vi "Kwang Min IHC images.vi"() -> ()   [LabVIEW 2020]
uses:
  <vilib>/picture/picture.llb/Draw True-Color Pixmap.vi
panel:
  out "SUM":u32
  in  "Find blue\nobjects?":bool
  in  "Count cells?":bool
  out "#cells":u8
  in  "Min cell size":i16=5
  in  "BLUE treshold":u8=175
  in  "GREEN treshold":u8=173
  in  "RED treshold":u8=180
  out "residue":i32
  in  "Binning points":u16=1
  out "BLUE":u8[](array[numeric])
  out "GREEN":u8[](array[numeric])
  out "RED":u8[](array[numeric])
  out "min BLUE":u8
  out "max BLUE":u8
  out "min GREEN":u8
  out "max GREEN":u8
  out "min RED":u8
  out "max RED":u8
  in  "stop":bool
  in  "rect":T1={"left"=38, "top"=68, "right"=53, "bottom"=89}
  in  "subset rect":T1={"left"=0, "top"=0, "right"=100, "bottom"=100}
  out "size(s)":i32[](array[numeric])
  out "new picture":picture
  out "Mask":u8[][](graph)
  in  "path to JPEG file":path
  # "cyan\nparticles"
  # "red\nparticles"
  # "All"
  # "210\n240\n165"
  # "240\n245\n250"
  # "0\n255\n255"
  # "170\n163\n183"
  # "159-255\n153-236\n175-242"
  # "926x1716"
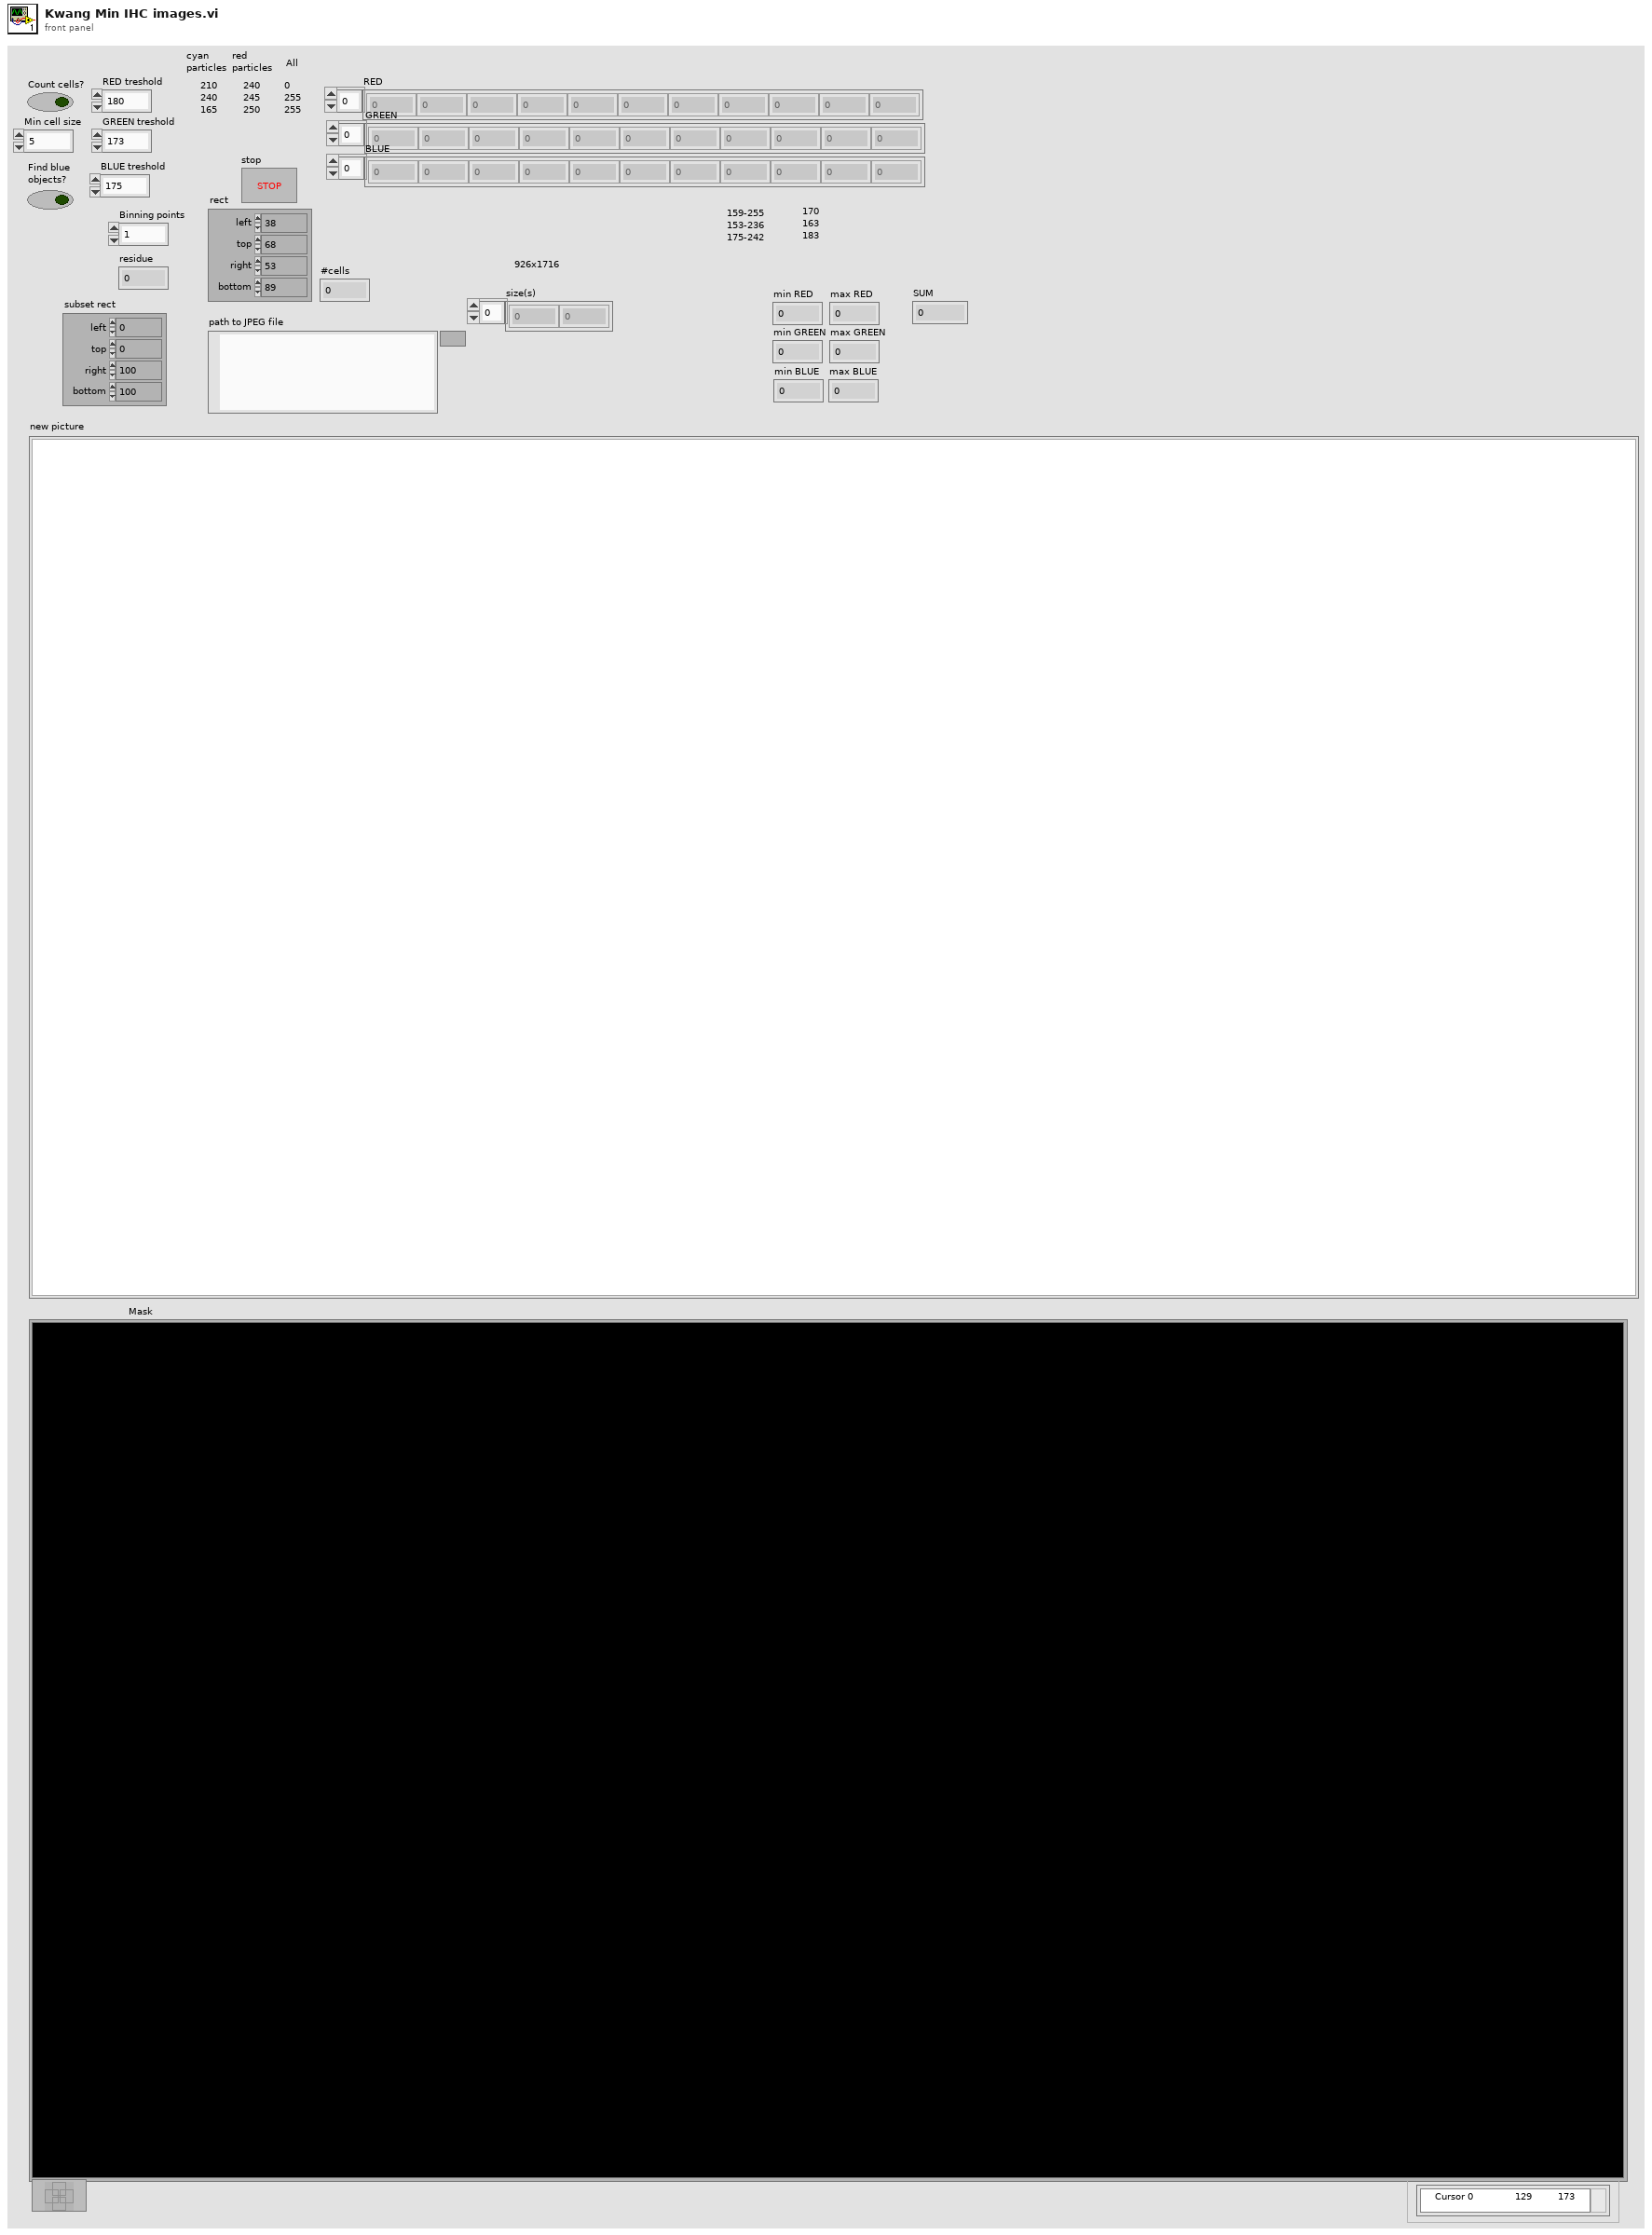
[diagram p1: front panel]
types:
  T1 = cluster{"left":i16, "top":i16, "right":i16, "bottom":i16}
  T2 = typedef "imagedata.ctl" = cluster{"image type":i32, "image depth":i32, "image":u8[], "mask":u8[], "colors":u32[], "Rectangle":cluster{"left":i16, "top":i16, "right":i16, "bottom":i16}}
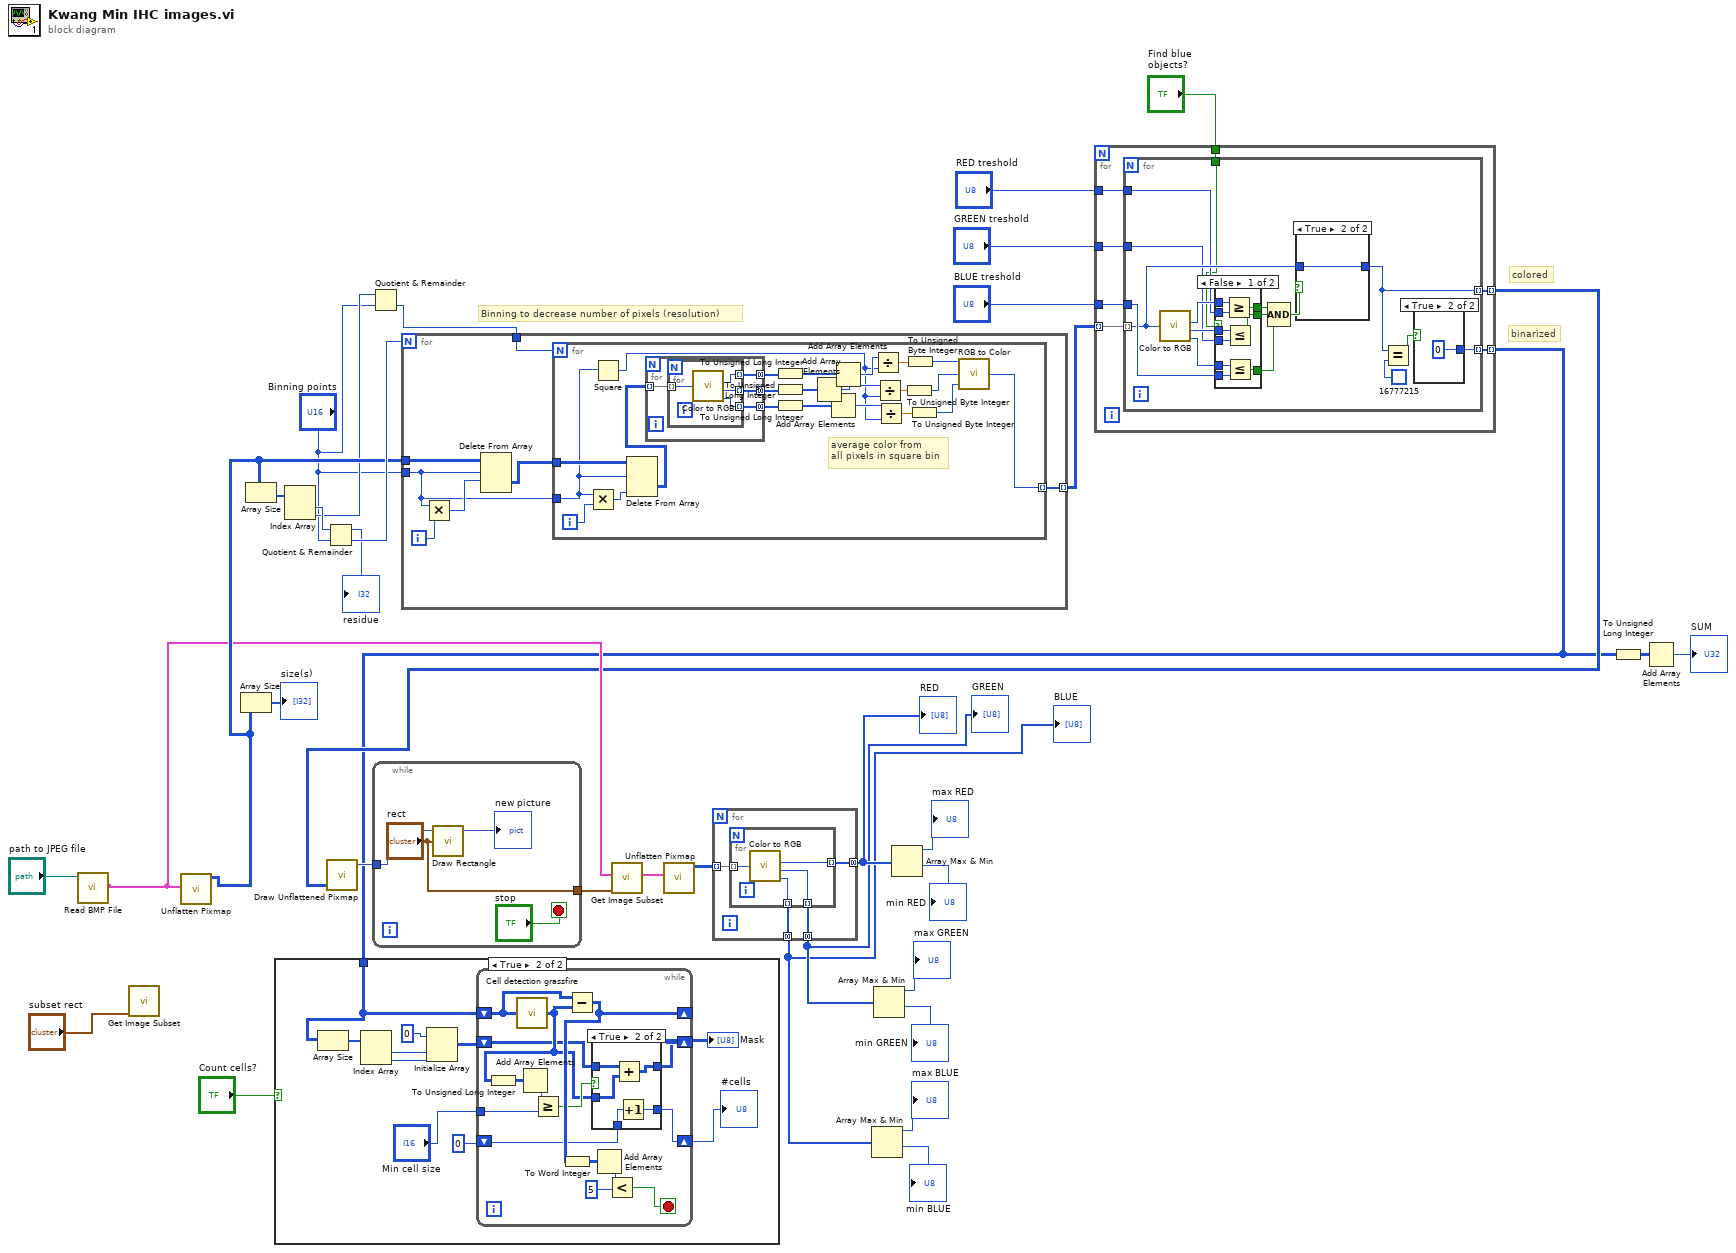
[diagram p0: block diagram]
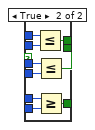
[diagram p4: hidden frame]
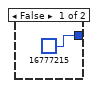
[diagram p5: hidden frame]
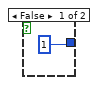
[diagram p6: hidden frame]
diagram:
  # "colored"
  # "binarized"
  # "Binning to decrease number of pixels (resolution)"
  n1 = call <vilib>:"Read BMP File.vi"("path to BMP file"="path to JPEG file") -> ("image data"=w14:T2)  [unwired: 8 in, 2 out]
  n2 = call <vilib>:"Get Image Subset.vi"("subset rect"="subset rect") -> ()  [unwired: 5 in, 2 out]
  n3 = call <vilib>:"Unflatten Pixmap.vi"("image data"=w14) -> ("24-bit pixmap"=w15:u32[][])  [unwired: 4 in, 6 out]
  n4 = Array Size(array=w15) -> (size(s)=→"size(s)":i32[])
  n5 = Array Size(array=w15) -> (size(s)=w19:i32[])
  n6 = Index Array(array=w19) -> (element #1=w18:i32, element #2=w13:i32)  [unwired: 2 in]
  n7 = Quotient & Remainder(x=w18, y="Binning points") -> (x-y*floor(x/y)=→"residue":i32, floor(x/y)=w17:i32)
  n8 = Quotient & Remainder(x=w13, y="Binning points") -> (floor(x/y)=w11:i32)  [unwired: 1 out]
  n9 = for {
    N: w17 -> [_]
    tunnel: w15 -> [w42]
    tunnel: "Binning points" -> [w37]
    tunnel: w11 -> [w38]
    tunnel: [w36] -> w10 mode=indexing
    i -> [w41]
    n10 = Multiply(x=w37, y=w41) -> (x*y=w40:i32)
    n11 = Delete From Array(array=w42, length=w37, index (row)=w40) -> (deleted portion=w39:u32[][])  [unwired: 1 in, 1 out]
    n12 = for {
      N: w38 -> [_]
      tunnel: w39 -> [w64]
      tunnel: w37 -> [w46]
      tunnel: [w49] -> w36 mode=indexing
      i -> [w62]
      # "average color from\nall pixels in square bin"
      n13 = Multiply(x=w46, y=w62) -> (x*y=w63:i32)
      n14 = Square(x=w46) -> (x^2=w47:u16)
      n15 = Delete From Array(array=w64, length=w46, index (col)=w63) -> (deleted portion=w61:u32[][])  [unwired: 1 in, 1 out]
      n16 = for {
        tunnel: w61 -> [w68] mode=indexing
        tunnel: [w67] -> w60 mode=concatenating
        tunnel: [w66] -> w59 mode=concatenating
        tunnel: [w65] -> w58 mode=concatenating
        n17 = for {
          tunnel: w68 -> [w72] mode=indexing
          tunnel: [w71] -> w67 mode=indexing
          tunnel: [w70] -> w66 mode=indexing
          tunnel: [w69] -> w65 mode=indexing
          n18 = call <vilib>:"Color to RGB.vi"("Color"=w72) -> ("R"=w71:u8, "G"=w70:u8, "B"=w69:u8)  [unwired: 1 out]
        }
      }
      n19 = To Unsigned Long Integer(number=w60) -> (unsigned 32bit integer=w57:u32[])
      n20 = To Unsigned Long Integer(number=w59) -> (unsigned 32bit integer=w56:u32[])
      n21 = To Unsigned Long Integer(number=w58) -> (unsigned 32bit integer=w55:u32[])
      n22 = Add Array Elements(numeric array=w56) -> (sum=w53:u32)
      n23 = Add Array Elements(numeric array=w55) -> (sum=w52:u32)
      n24 = Add Array Elements(numeric array=w57) -> (sum=w54:u32)
      n25 = Divide(x=w54, y=w47) -> (x/y=w51:dbl)
      n26 = Divide(x=w53, y=w47) -> (x/y=w50:dbl)
      n27 = Divide(x=w52, y=w47) -> (x/y=w48:dbl)
      n28 = To Unsigned Byte Integer(number=w50) -> (unsigned 8bit integer=w44:u8)
      n29 = To Unsigned Byte Integer(number=w51) -> (unsigned 8bit integer=w45:u8)
      n30 = To Unsigned Byte Integer(number=w48) -> (unsigned 8bit integer=w43:u8)
      n31 = call <vilib>:"RGB to Color.vi"("B"=w43, "G"=w44, "R"=w45) -> ("Color"=w49:u32)
    }
  }
  n32 = for {
    tunnel: w10 -> [w79] mode=indexing
    tunnel: "GREEN treshold" -> [w75]
    tunnel: "BLUE treshold" -> [w78]
    tunnel: [w77] -> w7 mode=indexing
    tunnel: [w76] -> w3 mode=indexing
    tunnel: "RED treshold" -> [w74]
    tunnel: "Find blue\nobjects?" -> [w73]
    n33 = for {
      tunnel: w79 -> [w91] mode=indexing
      tunnel: w78 -> [w95]
      tunnel: [w88] -> w77 mode=indexing
      tunnel: [w87] -> w76 mode=indexing
      tunnel: w75 -> [w86]
      tunnel: w74 -> [w85]
      tunnel: w73 -> [w80]
      n34 = call <vilib>:"Color to RGB.vi"("Color"=w91) -> ("R"=w94:u8, "G"=w93:u8, "B"=w92:u8)  [unwired: 1 out]
      n35 = case shown="False" w80 {
        tunnel: w95 -> [w103 w113]
        tunnel: w94 -> [w97 w112]
        tunnel: w93 -> [w100 w111]
        tunnel: w92 -> [w104 w110]
        tunnel: w86 -> [w99 w109]
        tunnel: w85 -> [w96 w108]
        tunnel: [w102 w107] -> w83
        tunnel: [w101 w106] -> w82
        tunnel: [w98 w105] -> w81
        frame False {
          n36 = Greater Or Equal?(x=w97, y=w96) -> (x >= y?=w98:bool)
          n37 = Less Or Equal?(x=w100, y=w99) -> (x <= y?=w101:bool)
          n38 = Less Or Equal?(x=w104, y=w103) -> (x <= y?=w102:bool)
        }
        frame True {
          n39 = Less Or Equal?(x=w112, y=w108) -> (x <= y?=w105:bool)
          n40 = Less Or Equal?(x=w111, y=w109) -> (x <= y?=w106:bool)
          n41 = Greater Or Equal?(x=w110, y=w113) -> (x >= y?=w107:bool)
        }
      }
      n42 = Compound Arithmetic op=AND(w81, w82, w83) -> (w84:bool)
      n43 = case shown="True" w84 {
        tunnel: w91 -> [_ w115]
        tunnel: [u32 16777215 ("Color") w115] -> w88
        frame False {
        }
        frame True {
        }
      }
      n44 = Equal?(x=w88, y=u32 16777215 ("Color")) -> (x = y?=w89:bool)
      n45 = case shown="True" w89 {
        tunnel: [u8 1 ("BLUE treshold") u8 0 ("BLUE treshold")] -> w87
        frame False {
        }
        frame True {
        }
      }
    }
  }
  n46 = case shown="True" "Count cells?" {
    tunnel: w3 -> [_ w126]
    frame False {
    }
    frame True {
      n47 = Array Size(array=w126) -> (size(s)=w125:i32[])
      n48 = Index Array(array=w125) -> (element #1=w124:i32, element #2=w123:i32)  [unwired: 2 in]
      n49 = Initialize Array(u8 0 ("BLUE treshold"), w124, w123) -> (w122:u8[][])
      n50 = while {
        shift-right: [w138] -> _
        shift-left: w126 -> [w142]
        shift-right: [w131] -> w121
        shift-left: w122 -> [w132]
        tunnel: "Min cell size" -> [w130]
        shift-right: [w129] -> w119
        shift-left: u8 0 ("BLUE treshold") -> [w128]
        stop <- w137 stop-if-true
        n51 = call "Cell detection grassfire.vi"("Intensities"=w142) -> ("Cell"=w133:u8[][])
        n52 = To Unsigned Long Integer(number=w133) -> (unsigned 32bit integer=w135:u32[][])
        n53 = Add Array Elements(numeric array=w135) -> (sum=w136:u32)
        n54 = Greater Or Equal?(x=w136, y=w130) -> (x >= y?=w134:bool)
        n55 = Subtract(x=w142, y=w133) -> (x-y=w138:u8[][])
        n56 = To Word Integer(number=w138) -> (16bit integer=w139:i16[][])
        n57 = case shown="True" w134 {
          tunnel: w133 -> [_ w149]
          tunnel: w132 -> [w144 w148]
          tunnel: [w144 w147] -> w131
          tunnel: [w143 w146] -> w129
          tunnel: w128 -> [w143 w145]
          frame False {
          }
          frame True {
            n58 = Add(x=w148, y=w149) -> (x+y=w147:u8[][])
            n59 = Increment(x=w145) -> (x+1=w146:u8)
          }
        }
        n60 = Add Array Elements(numeric array=w139) -> (sum=w141:i16)
        n61 = Less?(x=w141, y=i16 5) -> (x < y?=w137:bool)
      }
      "Mask" <- w121
      "#cells" <- w119
    }
  }
  n62 = call-poly <vilib>:"Draw Unflattened Pixmap.vi"("data (RGB format)"=w7) -> ("new picture"=w32:picture)  [unwired: 8 in]
  n63 = while {
    tunnel: w32 -> [w153]
    tunnel: ["rect"] -> w31
    stop <- "stop" stop-if-true
    n64 = call <vilib>:"Draw Rectangle.vi"("picture"=w153, "rect"="rect") -> ("new picture"=→"new picture":picture)  [unwired: 7 in]
  }
  n65 = call <vilib>:"Get Image Subset.vi"("subset rect"=w31, "image data"=w14) -> ("image subset"=w30:T2)  [unwired: 4 in, 1 out]
  n66 = call <vilib>:"Unflatten Pixmap.vi"("image data"=w30) -> ("24-bit pixmap"=w29:u32[][])  [unwired: 4 in, 6 out]
  n67 = for {
    tunnel: w29 -> [w157] mode=indexing
    tunnel: [w156] -> w22 mode=concatenating
    tunnel: [w155] -> w21 mode=concatenating
    tunnel: [w154] -> w20 mode=concatenating
    n68 = for {
      tunnel: w157 -> [w161] mode=indexing
      tunnel: [w160] -> w156 mode=indexing
      tunnel: [w159] -> w155 mode=indexing
      tunnel: [w158] -> w154 mode=indexing
      n69 = call <vilib>:"Color to RGB.vi"("Color"=w161) -> ("R"=w160:u8, "G"=w159:u8, "B"=w158:u8)  [unwired: 1 out]
    }
  }
  "RED" <- w22
  "GREEN" <- w21
  "BLUE" <- w20
  n70 = Array Max & Min(array=w20) -> (max value=→"max BLUE":u8, min value=→"min BLUE":u8)  [unwired: 2 out]
  n71 = Array Max & Min(array=w21) -> (max value=→"max GREEN":u8, min value=→"min GREEN":u8)  [unwired: 2 out]
  n72 = Array Max & Min(array=w22) -> (max value=→"max RED":u8, min value=→"min RED":u8)  [unwired: 2 out]
  n73 = To Unsigned Long Integer(number=w3) -> (unsigned 32bit integer=w2:u32[][])
  n74 = Add Array Elements(numeric array=w2) -> (sum=→"SUM":u32)
